vi "Assign Placeholder Data to match SP4T.vi"(7 "SP4T_Pins":string[](array[string]), 8 "error in (no error)":errorcluster, 10 "Individual_R_Meas":dbl[](array[numeric]), 11 "USID":T1 max=15) -> (0 "error out":errorcluster, 3 "Placeholder_w_Data":dbl[](array[numeric]))   [LabVIEW 2013]
uses:
  Controls/USID.ctl
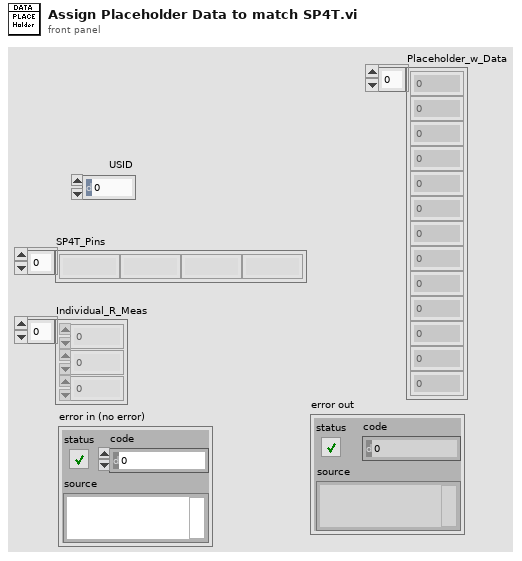
[diagram p1: front panel]
types:
  T1 = typedef "USID.ctl" = u8
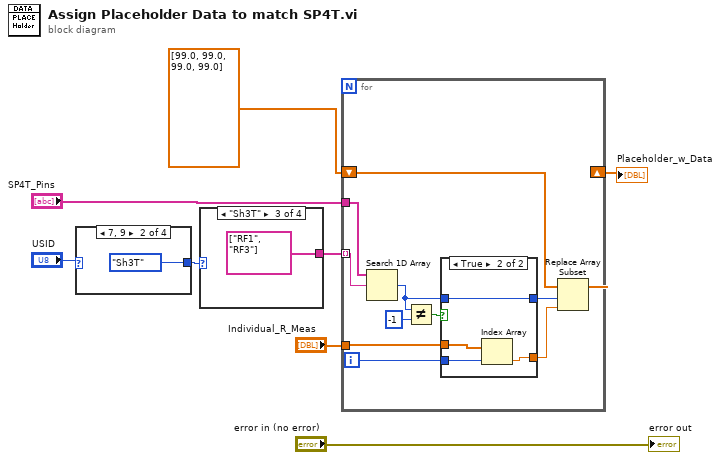
[diagram p0: block diagram]
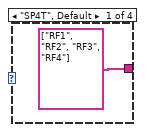
[diagram p2: hidden frame]
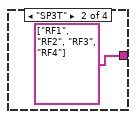
[diagram p3: hidden frame]
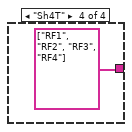
[diagram p4: hidden frame]
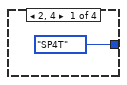
[diagram p5: hidden frame]
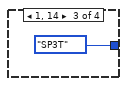
[diagram p6: hidden frame]
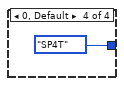
[diagram p7: hidden frame]
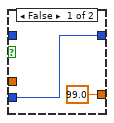
[diagram p8: hidden frame]
diagram:
  n1 = case shown="7, 9" "USID" {
    tunnel: [enum16{"SP4T", "SP3T", "Sh3T", "Sh4T"}."SP4T" ("Die Type 2") enum16{"SP4T", "SP3T", "Sh3T", "Sh4T"}."Sh3T" ("Die Type 2") enum16{"SP4T", "SP3T", "Sh3T", "Sh4T"}."SP3T" ("Die Type 2") enum16{"SP4T", "SP3T", "Sh3T", "Sh4T"}."SP4T" ("Die Type 2")] -> w2
    frame 2, 4 {
    }
    frame 7, 9 {
    }
    frame 1, 14 {
    }
    frame 0, Default {
    }
  }
  n2 = case shown="\"Sh3T\"" w2 {
    tunnel: [string[] ["RF1", "RF2", "RF3", "RF4"] string[] ["RF1", "RF2", "RF3", "RF4"] string[] ["RF1", "RF3"] string[] ["RF1", "RF2", "RF3", "RF4"]] -> w1
    frame "SP4T", Default {
    }
    frame "SP3T" {
    }
    frame "Sh3T" {
    }
    frame "Sh4T" {
    }
  }
  n3 = for {
    tunnel: "Individual_R_Meas" -> [w27]
    tunnel: "SP4T_Pins" -> [w18]
    shift-right: [w24] -> w3
    shift-left: dbl[] [99.0, 99.0, 99.0, 99.0] ("Placeholder_w_Data") -> [w25]
    tunnel: w1 -> [w17] mode=indexing
    i -> [w26]
    n4 = Search 1D Array(1D array=w18, element=w17) -> (index of element=w21:i32)  [unwired: 1 in]
    n5 = Not Equal?(x=w21, y=-1) -> (x != y?=w22:bool)
    n6 = case shown="True" w22 {
      tunnel: w27 -> [_ w33]
      tunnel: w21 -> [_ w31]
      tunnel: [99.0 w32] -> w20
      tunnel: w26 -> [w28 w30]
      tunnel: [w28 w31] -> w19
      frame False {
      }
      frame True {
        n7 = Index Array(array=w33, index=w30) -> (element=w32:dbl)
      }
    }
    n8 = Replace Array Subset(array=w25, new element=w20, index=w19) -> (w24:dbl[])
  }
  "Placeholder_w_Data" <- w3
  "error out" <- "error in (no error)"
